vi "ETHANOL.vi"() -> (3 "Numeric":dbl)   [LabVIEW 2021]
panel:
  out "error out":errorcluster
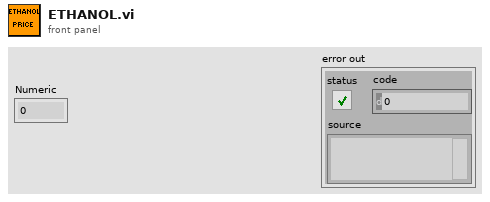
[diagram p1: front panel]
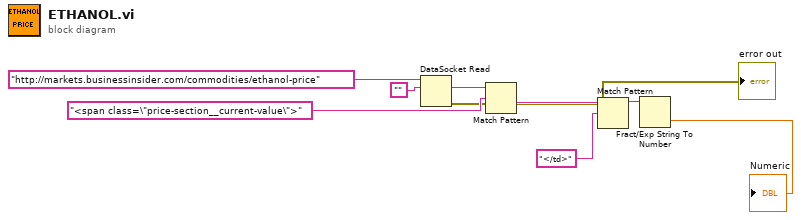
[diagram p0: block diagram]
diagram:
  n1 = DataSocket Read(10:"", 11:"http://markets.businessinsider.com/commodities/ethanol-price") -> (0:→"error out":errorcluster, 2:w4:string)  [unwired: 3 in, 5 out]
  n2 = Match Pattern(string=w4, regular expression="<span class=\"price-section__current-value\">") -> (after substring=w6:string)  [unwired: 1 in, 3 out]
  n3 = Match Pattern(string=w6, regular expression="</td>") -> (before substring=w8:string)  [unwired: 1 in, 3 out]
  n4 = Fract/Exp String To Number(string=w8) -> (number=→"Numeric":dbl)  [unwired: 3 in, 1 out]
